vi "Write to Lights.vi"   [LabVIEW 2015]
types:
  T1 = typedef "WPI_DriverStationRobotMode2.ctl" = enum16{"Autonomous Disabled", "Autonomous Enabled", "Teleop Disabled", "Teleop Enabled", "Disconnected", "Finish", "Test Disabled", "Test Enabled", "Emergency Stopped"}
  T2 = typedef "WPI_DigitalOutputDevRef.ctl" = cluster{"DIO Channel":T3, "DevStatus":errorcluster}
  T3 = typedef "FPGA_DIOChannel.ctl" = enum8{"DIO 0", "DIO 1", "DIO 2", "DIO 3", "DIO 4", "DIO 5", "DIO 6", "DIO 7", "DIO 8", "DIO 9", "DIO MXP 0", "DIO MXP 1", "DIO MXP 2", "DIO MXP 3", "DIO MXP 4", "DIO MXP 5", "DIO MXP 6", "DIO MXP 7", "DIO MXP 8", "DIO MXP 9", "DIO MXP 10", "DIO MXP 11", "DIO MXP 12", "DIO MXP 13", "DIO MXP 14", "DIO MXP 15", "Invalid"}
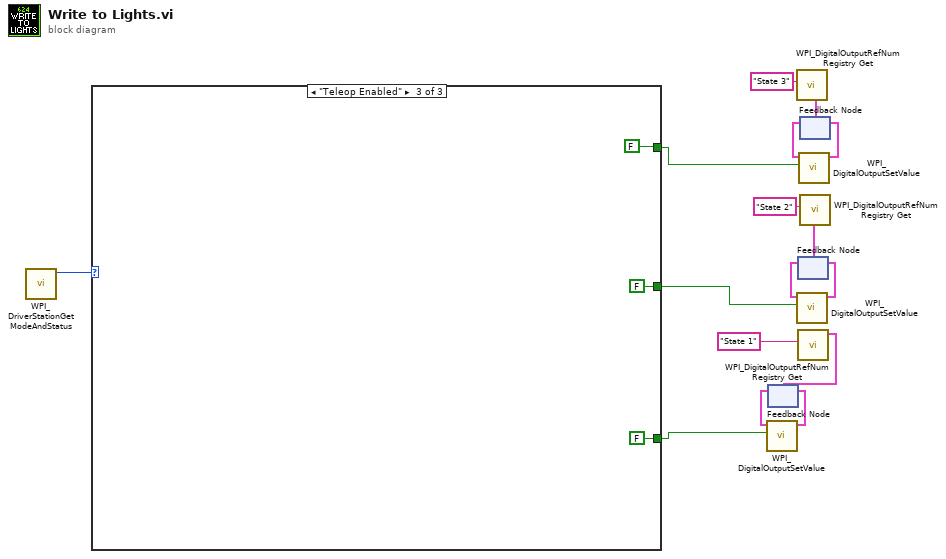
[diagram p0: block diagram]
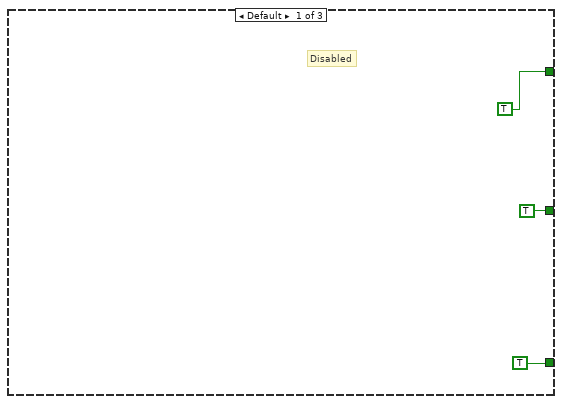
[diagram p2: hidden frame]
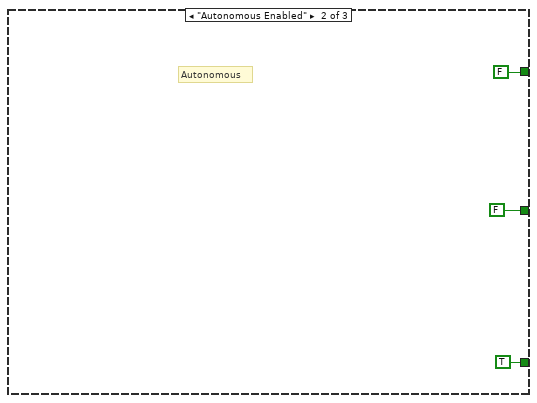
[diagram p3: hidden frame]
diagram:
  n1 = call <vilib>:"WPI_DriverStationGetModeAndStatus.vi"() -> ("Robot Mode"=w4:T1)  [unwired: 10 in, 1 out]
  n2 = case shown="\"Teleop Enabled\"" w4 {
    tunnel: [TRUE FALSE FALSE] -> w1
    tunnel: [TRUE FALSE FALSE] -> w2
    tunnel: [TRUE TRUE FALSE] -> w3
    frame Default {
      # "Disabled"
    }
    frame "Autonomous Enabled" {
      # "Autonomous"
    }
    frame "Teleop Enabled" {
    }
  }
  n3 = call <vilib>:"WPI_DigitalOutputRefNum Registry Get.vi"("refnum name"="State 3") -> ("DigitalOutputDevRef"=w9:T2)  [unwired: 9 in, 1 out]
  n4 = call <vilib>:"WPI_DigitalOutputRefNum Registry Get.vi"("refnum name"="State 1") -> ("DigitalOutputDevRef"=w5:T2)  [unwired: 9 in, 1 out]
  n5 = feedback #1(w5) -> (w14:T2)
  n6 = call <vilib>:"WPI_DigitalOutputSetValue.vi"("Value"=w3, "DigitalOutputDevRef"=w14) -> ("DigitalOutputDevRef"=w15:T2)  [unwired: 8 in, 1 out]
  n7 = feedback-in #1(w15) -> ()
  n8 = feedback #2(w9) -> (w8:T2)
  n9 = call <vilib>:"WPI_DigitalOutputSetValue.vi"("Value"=w1, "DigitalOutputDevRef"=w8) -> ("DigitalOutputDevRef"=w6:T2)  [unwired: 8 in, 1 out]
  n10 = feedback-in #2(w6) -> ()
  n11 = call <vilib>:"WPI_DigitalOutputRefNum Registry Get.vi"("refnum name"="State 2") -> ("DigitalOutputDevRef"=w10:T2)  [unwired: 9 in, 1 out]
  n12 = feedback #3(w10) -> (w12:T2)
  n13 = call <vilib>:"WPI_DigitalOutputSetValue.vi"("Value"=w2, "DigitalOutputDevRef"=w12) -> ("DigitalOutputDevRef"=w11:T2)  [unwired: 8 in, 1 out]
  n14 = feedback-in #3(w11) -> ()
